vi "auto_sl.vi"() -> ()   [LabVIEW 2012, in "Serenity_mk2.lvrbt"]
uses:
  Serenity_mk2.lvrbt
  MecanumDrive/Mecanum Drive.lvrbt
  <vilib>/NXT/Hardware/Plugins/Tetrix DC Motor/TetrixDCMotorAddress.ctl
  <vilib>/NXT/LegoClasses/BrickReference/BrickReference.lvclass
  <vilib>/NXT/Subs/LVHSConnector.ctl
  <vilib>/NXT/NXTIO Xnodes/NXTIONodeSubVIs/TETRIX IO Stop DC Motors.vi
  <vilib>/NXT/NXTIO Xnodes/NXTIOXNode/NXTIO.xnode
  <vilib>/NXT/NXTIO Xnodes/AddressXNode/NXTIOAddress.xnode
  <vilib>/NXT/Block Support/NXT_InputPort.ctl
  <vilib>/NXT/HiTechnic/HiTechnic Controls/HiTechnic Port.ctl
  Serenity_mk2/SubVIs/State_Typ.ctl
  Serenity_mk2/SubVIs/auto_drive_TYP.ctl
  <vilib>/NXT/Dual Mode Library/Sound/Tone.vi
  <vilib>/NXT/Dual Mode Library/Waits/Wait_Num.vi
  <vilib>/NXT/Dual Mode Library/Display/drawNumber.vi
  <vilib>/NXT/Dual Mode Library/Waits/Wait_Num(msec).vi
  <vilib>/NXT/NXTIO Xnodes/NXTIONodeSubVIs/TETRIX IO Check Battery.vi
  <vilib>/NXT/NXTIO Xnodes/NXTIONodeSubVIs/TETRIX IO Reset Encoders.vi
  <vilib>/NXT/NXTIO Xnodes/NXTIONodeSubVIs/TETRIX IO Motor Status.vi
  <vilib>/NXT/Hardware/Plugins/Tetrix 180 deg Servo/Tetrix180ServoAddress.ctl
  <vilib>/NXT/NXTIO Xnodes/NXTIONodeSubVIs/TETRIX IO Move Servos.vi
panel:
  out "Enabled":bool
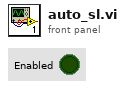
[diagram p1: front panel]
types:
  T1 = typedef "auto_drive_TYP.ctl" = cluster{"Left X":i8, "Left Y":i8, "Right X":i8, "Power (100)":i8, "Wait (ms)":u32, "Enc/Deg Target":i32, "Move Type":enum16{"Relative Degrees", "Wait", "Encoder"}}
  T2 = typedef "State_Typ.ctl" = enum16{"Stop", "Check for Position 3", "Check for Position 2", "Move", "Reset Enc", "Read Enc"}
  T3 = typedef "HiTechnic Port.ctl" = cluster{"Port":T4, "MUX Port":u8}
  T4 = typedef "NXT_InputPort.ctl" = u32
  T5 = typedef "TetrixDCMotorAddress.ctl" = i32
  T6 = typedef "LVHSConnector.ctl" = refnum<class "BrickReference.lvclass">
  T7 = typedef "Tetrix180ServoAddress.ctl" = i32
  T8 = cluster{"TetrixDCMotor":T5, "TetrixDCMotor 2":T5}
  T9 = cluster{"Direction (0-9)":i16, "Signal Strength (Array)":u8[]}
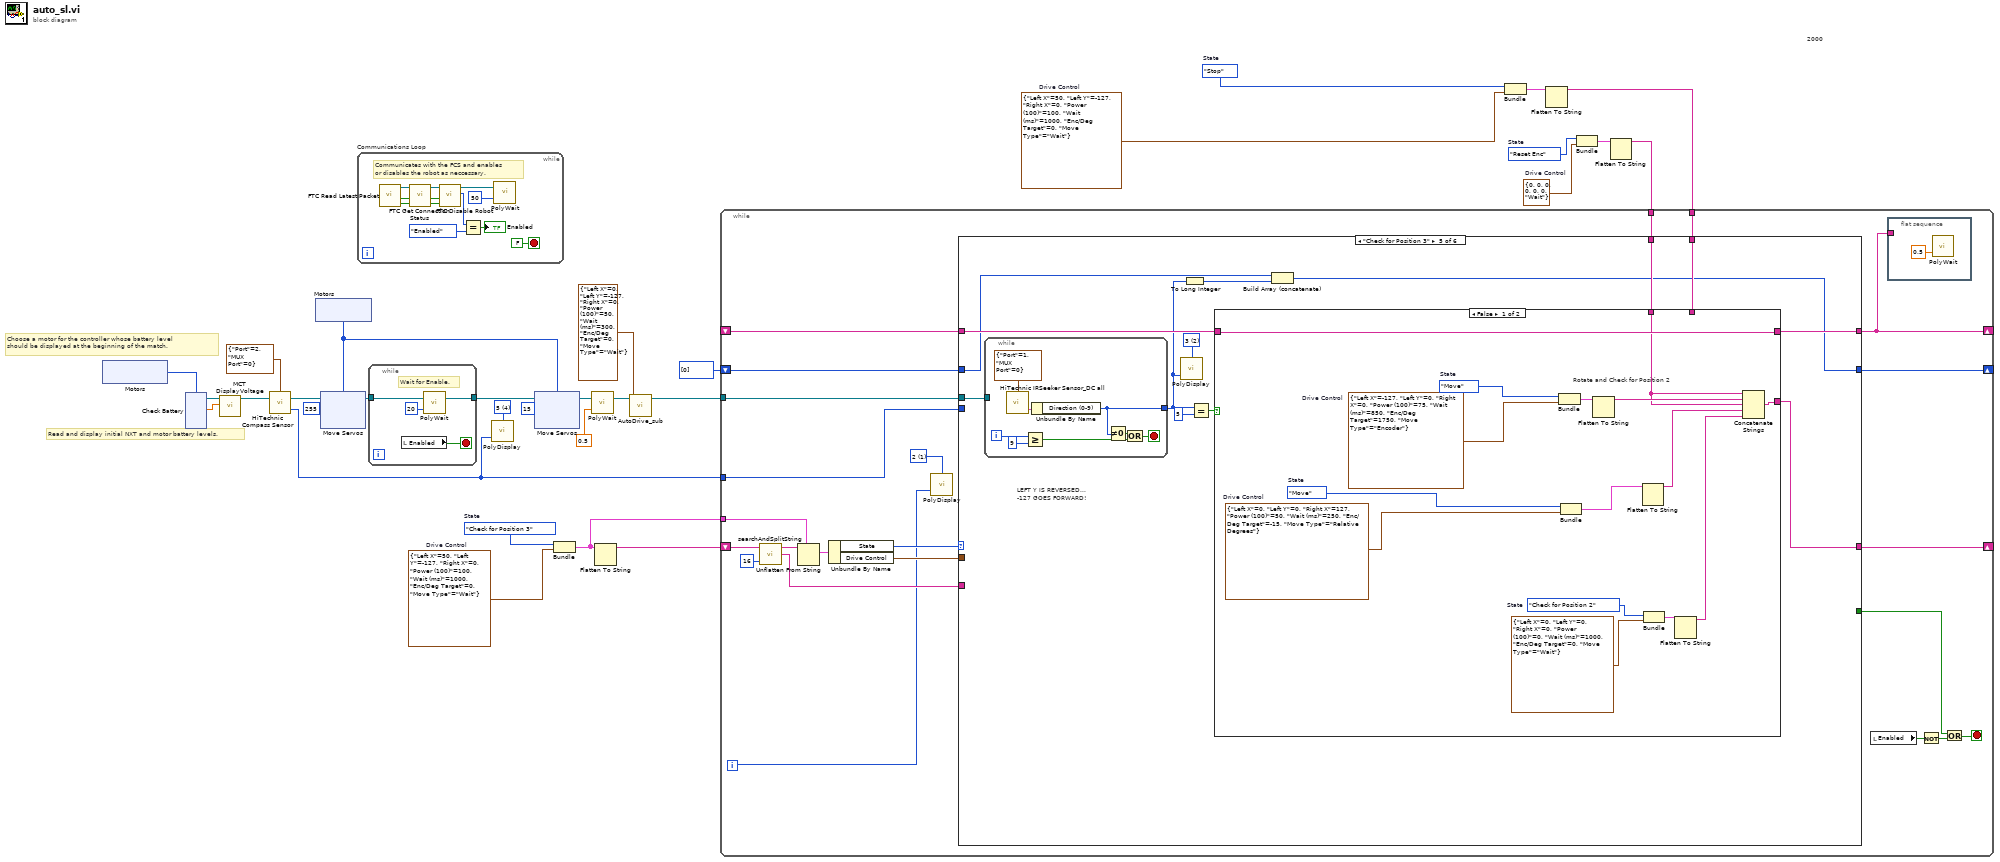
[diagram p0: block diagram]
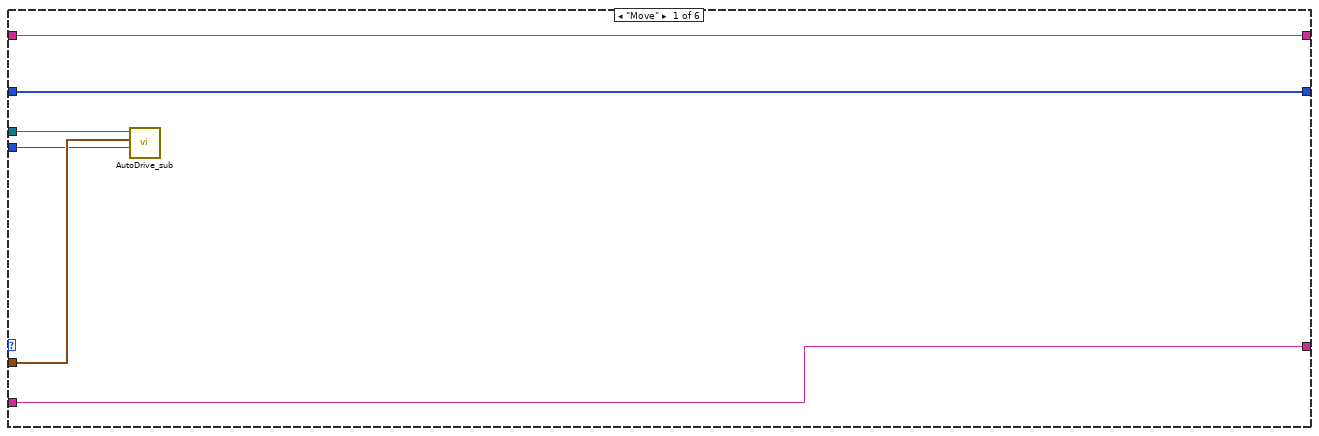
[diagram p2: hidden frame]
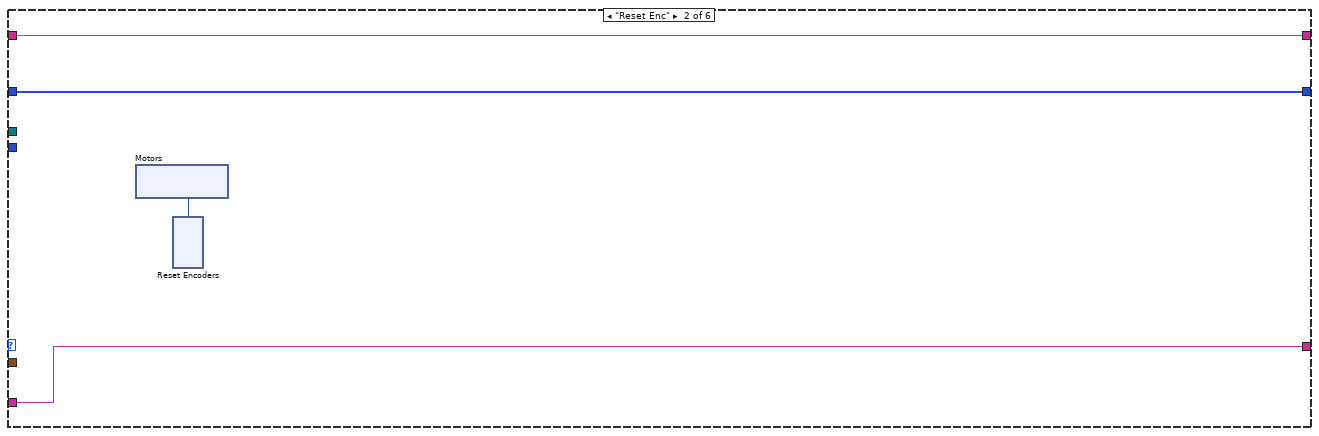
[diagram p3: hidden frame]
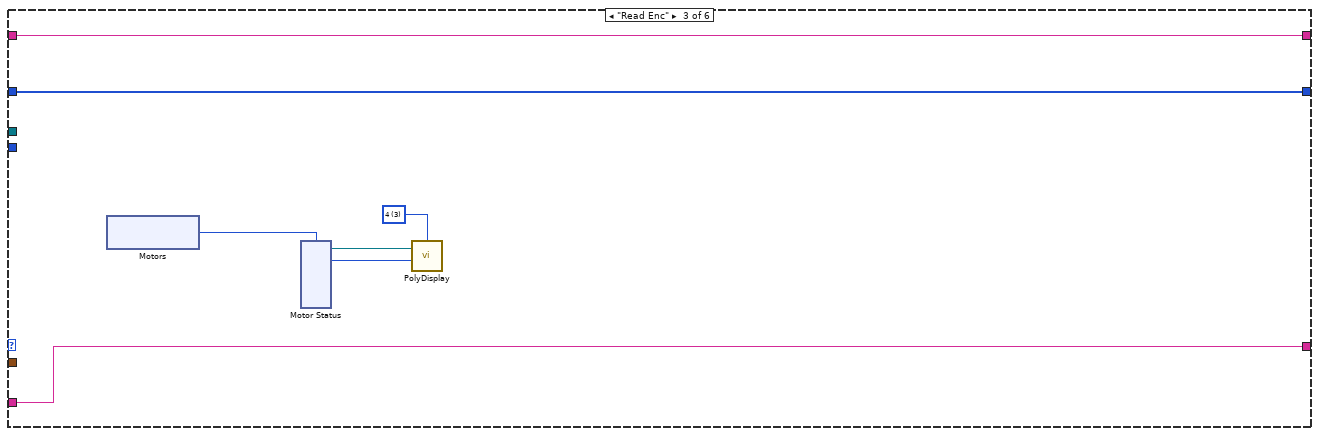
[diagram p4: hidden frame]
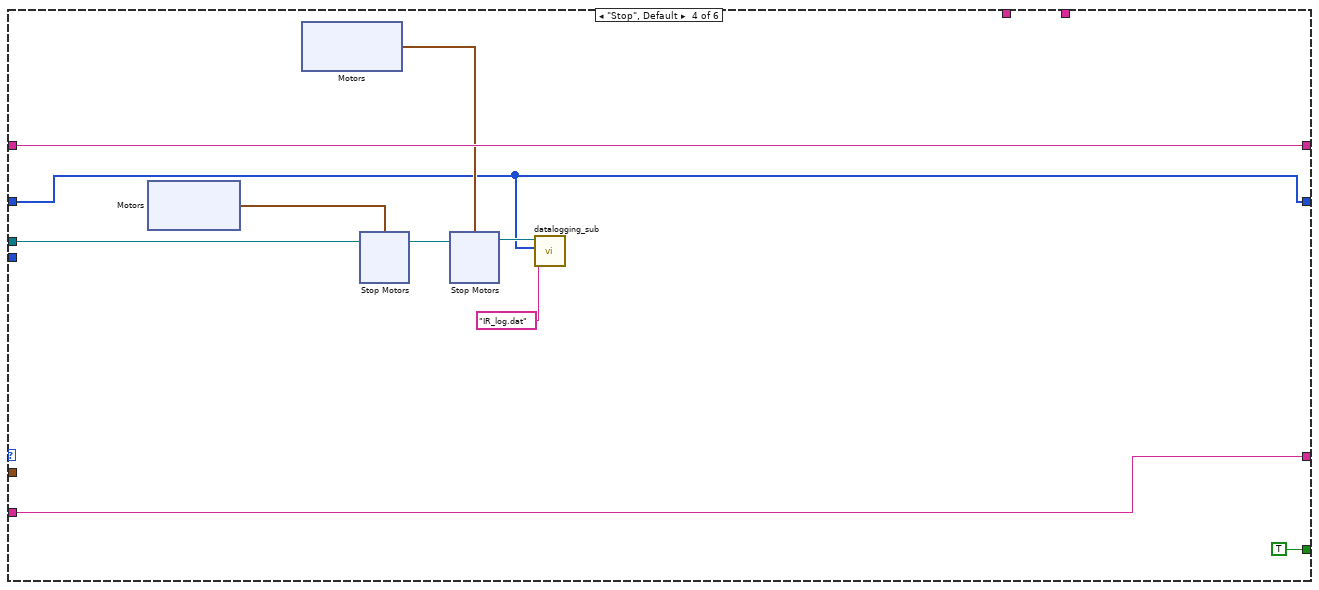
[diagram p5: hidden frame]
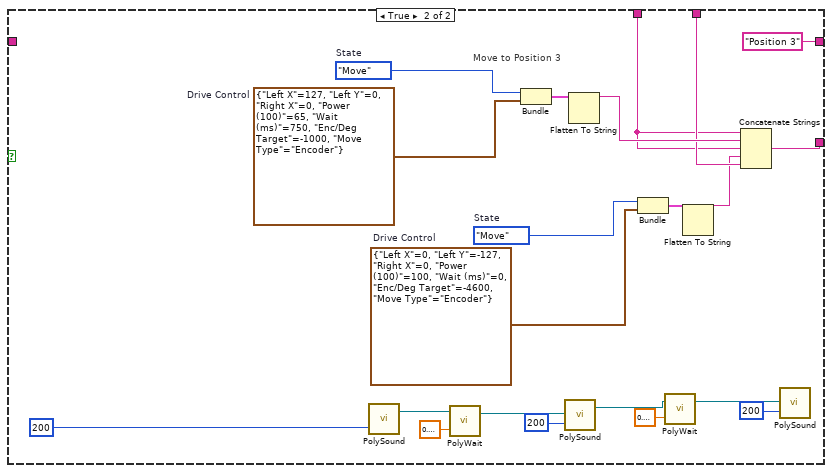
[diagram p6: hidden frame]
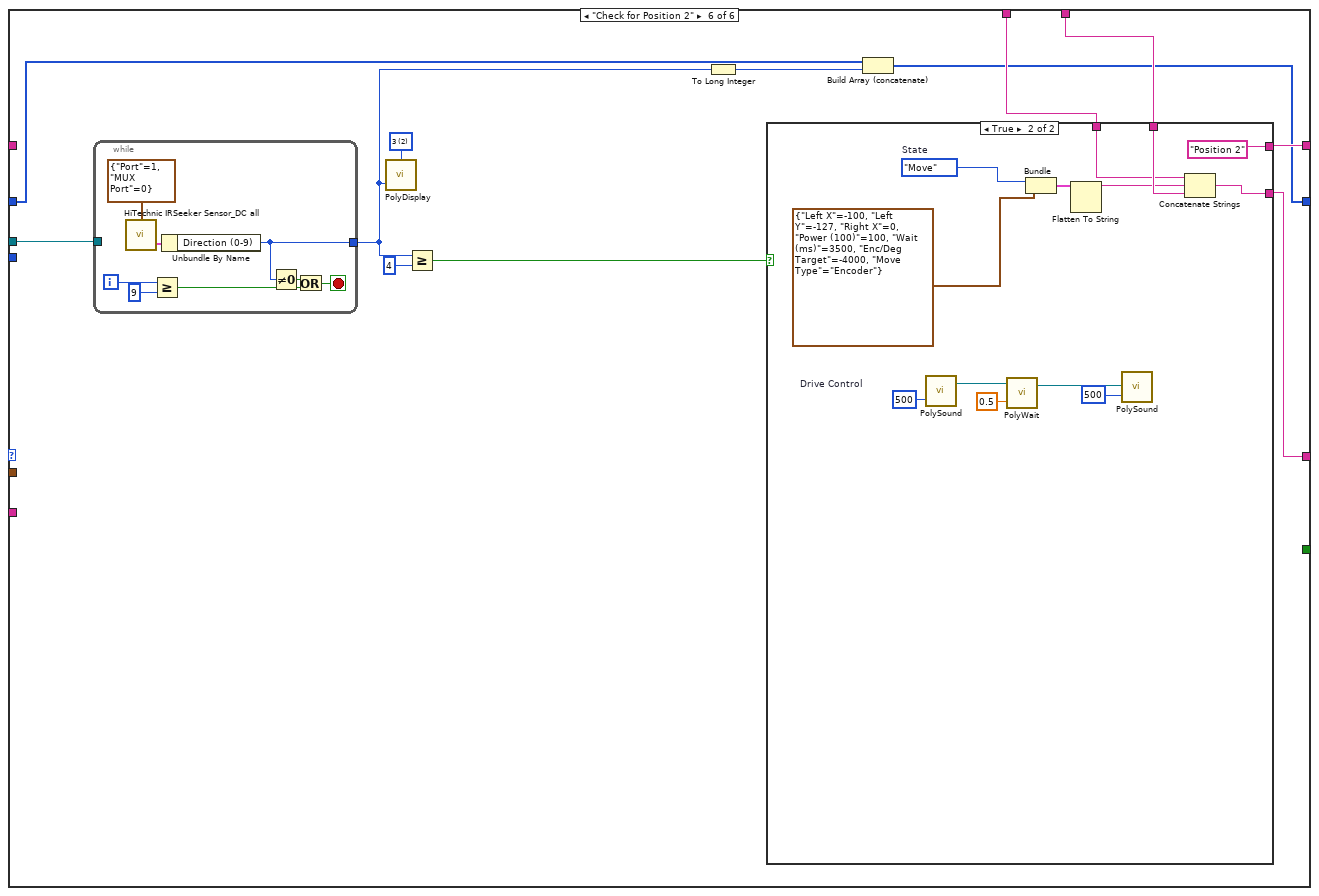
[diagram p7: hidden frame]
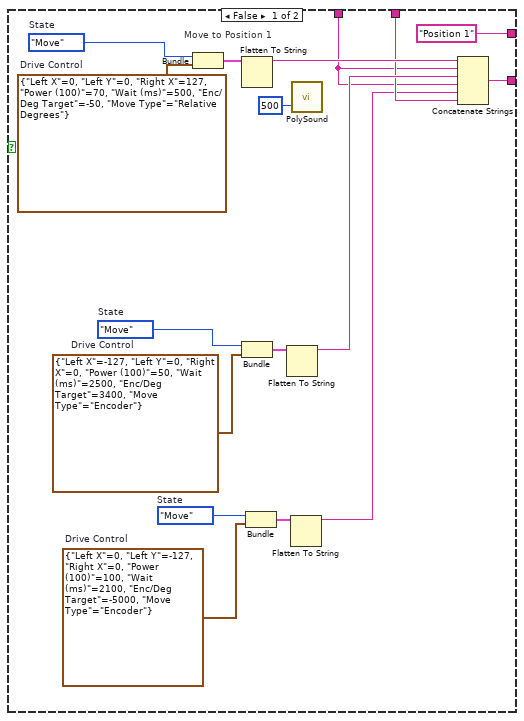
[diagram p8: hidden frame]
diagram:
  w11 = T1 {"Left X"=0, "Left Y"=0, "Right X"=0, "Power (100)"=0, "Wait (ms)"=0, "Enc/Deg Target"=0, "Move Type"=enum."Wait"}  # Drive Control
  w13 = State_Typ."Reset Enc"  # State
  w18 = T1 {"Left X"=50, "Left Y"=-127, "Right X"=0, "Power (100)"=100, "Wait (ms)"=1000, "Enc/Deg Target"=0, "Move Type"=enum."Wait"}  # Drive Control
  w19 = State_Typ."Stop"  # State
  w22 = i16 4 items=["1", "2", "3", "4", "5", "6", "7", "8", "9", "10", "11", "12"] ("Line")
  w31 = T1 {"Left X"=50, "Left Y"=-127, "Right X"=0, "Power (100)"=100, "Wait (ms)"=1000, "Enc/Deg Target"=0, "Move Type"=enum."Wait"}  # Drive Control
  w30 = State_Typ."Check for Position 3"  # State
  # "2000"
  # "Read and display initial NXT and motor battery levels."
  # "Choose a motor for the controller whose battery level \nshould be displayed at the beginning of the match."
  n1 = xnode "Motors"() -> ("Motor"=w27:T5)
  n2 = xnode "Check Battery"("Motors"=w27) -> ("Voltage 1"=w28:sgl, "NXT/EV3"=w29:T6)  [unwired: 1 in]
  n3 = call <vilib>:"MCT DisplayVoltage.vi"("Motor Voltage"=w28, "NXT"=w29) -> ("NXT"=w23:T6)  [unwired: 9 in]
  n4 = call <vilib>:"HiTechnic Compass Sensor.vi"("NXT/EV3"=w23, "Port/MUX"=T3 {"Port"=2, "MUX Port"=0}) -> ("Heading (degrees)"=w21:i16, "NXT/EV3"=w10:T6)  [unwired: 1 in]
  n5 = xnode "Motors"() -> ("Motor"=w6:T7)
  n6 = xnode "Move Servos"("Position 1"=u8 255, "Motors"=w6, "NXT/EV3"=w10) -> ("NXT/EV3"=w9:T6)
  n7 = while "Communications Loop" {
    stop <- FALSE stop-if-true
    # "Communicates with the FCS and enables \nor disables the robot as neccessary."
    n8 = call <vilib>:"FTC Read Latest Packet.vi"() -> ("Packet Received?"=w41:bool, "Stopped?"=w40:bool, "NXT"=w43:T6)  [unwired: 6 in, 3 out]
    n9 = call <vilib>:"FTC Get Connection Status.vi"("Packet Received?"=w41, "Stopped?"=w40, "NXT"=w43) -> ("Online?"=w32:bool, "Stopped?"=w33:bool, "NXT"=w42:T6)  [unwired: 5 in]
    n10 = call <vilib>:"FTC Disable Robot.vi"("Online?"=w32, "Stopped?"=w33, "NXT"=w42) -> ("Enabled?"=w36:enum16{"Disabled", "Enabled"}, "NXT"=w38:T6)  [unwired: 3 in]
    n11 = Equal?(x=w36, y=enum16{"Disabled", "Enabled"}."Enabled") -> (x = y?=→"Enabled":bool)
    n12 = call-poly <vilib>:"PolyWait.vi"("Time (100 msec)"=u32 50 ("Time (msec)"), "NXT/EV3"=w38) -> ()  [unwired: 2 in, 1 out]
  }
  n13 = while {
    tunnel: [w45] -> w5
    tunnel: w9 -> [w44]
    stop <- w46 stop-if-true
    # "Wait for Enable."
    n14 = local read "Enabled"() -> (w46:bool)
    n15 = call-poly <vilib>:"PolyWait.vi"("Time (100 msec)"=u32 20 ("Time (msec)"), "NXT/EV3"=w44) -> ("NXT/EV3"=w45:T6)  [unwired: 2 in]
  }
  n16 = call-poly <vilib>:"PolyDisplay.vi"("number"=w21, "Line"=w22) -> ()  [unwired: 2 in, 1 out]
  n17 = xnode "Move Servos"("Position 1"=u8 15, "Motors"=w6, "NXT/EV3"=w5) -> ("NXT/EV3"=w2:T6)
  n18 = Bundle("State"=w30, "Drive Control"=w31) -> (w26:cluster{"State":T2, "Drive Control":T1})  [unwired: 1 in]
  n19 = call-poly <vilib>:"PolyWait.vi"("Time (1 sec)"=sgl 0.5, "NXT/EV3"=w2) -> ("NXT/EV3"=w3:T6)  [unwired: 2 in]
  n20 = Flatten To String(anything=w26) -> (data string=w25:string)  [unwired: 3 in, 2 out]
  n21 = call "AutoDrive_sub.vi"("Drive Control"=T1 {"Left X"=0, "Left Y"=-127, "Right X"=0, "Power (100)"=50, "Wait (ms)"=300, "Enc/Deg Target"=0, "Move Type"=enum."Wait"}, "NXT/EV3"=w3) -> ("NXT/EV3 out"=w7:T6)  [unwired: 8 in, 1 out]
  n22 = Bundle("State"=w19, "Drive Control"=w18) -> (w20:cluster{"State":T2, "Drive Control":T1})  [unwired: 1 in]
  n23 = Flatten To String(anything=w20) -> (data string=w17:string)  [unwired: 3 in, 2 out]
  n24 = Bundle("State"=w13, "Drive Control"=w11) -> (w14:cluster{"State":T2, "Drive Control":T1})  [unwired: 1 in]
  n25 = Flatten To String(anything=w14) -> (data string=w12:string)  [unwired: 3 in, 2 out]
  n26 = while {
    tunnel: w7 -> [w70]
    shift-right: [w61] -> _
    shift-left: w25 -> [w59]
    tunnel: w26 -> [w62]
    shift-right: [w52] -> _
    shift-left: _ -> [w60]
    tunnel: w17 -> [w57]
    tunnel: w21 -> [w51]
    shift-right: [w50] -> _
    shift-left: i32[] [0] -> [w49]
    tunnel: w12 -> [w48]
    i -> [w53]
    stop <- w69 stop-if-true
    w54 = i16 1 items=["1", "2", "3", "4", "5", "6", "7", "8", "9", "10", "11", "12"] ("Line")
    n27 = call <vilib>:"searchAndSplitString.vi"("offset (0)"=16 ("length (rest)"), "string"=w59) -> ("match + rest of string"=w58:string, "substring before match"=w64:string)  [unwired: 1 in, 1 out]
    n28 = Unflatten From String(type=w62, binary string=w64) -> (value=w63:cluster{"State":T2, "Drive Control":T1})  [unwired: 3 in, 2 out]
    n29 = Unbundle By Name(w63) -> ("State"=w55:T2, "Drive Control"=w65:T1)
    n30 = call-poly <vilib>:"PolyDisplay.vi"("number"=w53, "Line"=w54) -> ()  [unwired: 2 in, 1 out]
    n31 = case shown="\"Check for Position 3\"" w55 {
      tunnel: w70 -> [w77 _ _ w112 w125 w186]
      tunnel: [_ _ _ TRUE _ _] -> w68
      tunnel: w65 -> [w76 _ _ _ _ _]
      tunnel: w58 -> [w75 w81 w93 w110 _ _]
      tunnel: [w75 w81 w93 w110 w133 w191] -> w61
      tunnel: [w74 w80 w92 w109 w136 w193] -> w52
      tunnel: w60 -> [w74 w80 w92 w109 w135 _]
      tunnel: w57 -> [_ _ _ _ w134 w192]
      tunnel: w51 -> [w73 _ _ _ _ _]
      tunnel: [w72 w78 w87 w104 w128 w189] -> w50
      tunnel: w49 -> [w72 w78 w87 w104 w129 w188]
      tunnel: w48 -> [_ _ _ _ w130 w190]
      frame "Move" {
        n32 = call "AutoDrive_sub.vi"("Target Heading (Degrees)"=w73, "Drive Control"=w76, "NXT/EV3"=w77) -> ()  [unwired: 7 in, 2 out]
      }
      frame "Reset Enc" {
        n33 = xnode "Motors"() -> ("Motor"=w79:T5)
        n34 = xnode "Reset Encoders"("Motors"=w79) -> ()  [unwired: 1 in, 1 out]
      }
      frame "Read Enc" {
        w89 = i16 3 items=["1", "2", "3", "4", "5", "6", "7", "8", "9", "10", "11", "12"] ("Line")
        n35 = xnode "Motors"() -> ("Motor"=w91:T5)
        n36 = xnode "Motor Status"("Motors"=w91) -> ("Position 1"=w90:i32, "NXT/EV3"=w88:T6)  [unwired: 1 in, 1 out]
        n37 = call-poly <vilib>:"PolyDisplay.vi"("number"=w90, "NXT/EV3"=w88, "Line"=w89) -> ()  [unwired: 1 in, 1 out]
      }
      frame "Stop", Default {
        n38 = xnode "Motors"() -> ("Motor"=w108:cluster{"TetrixDCMotor":T5, "TetrixDCMotor":T5})
        n39 = xnode "Motors"() -> ("Motor"=w107:cluster{"TetrixDCMotor":T5, "TetrixDCMotor":T5})
        n40 = xnode "Stop Motors"("Motors"=w108, "NXT/EV3"=w112) -> ("NXT/EV3"=w106:T6)
        n41 = xnode "Stop Motors"("Motors"=w107, "NXT/EV3"=w106) -> ("NXT/EV3"=w105:T6)
        n42 = call "datalogging_sub.vi"("Path Selected"="IR_log.dat" ("Filename"), "States Executed"=w104, "NXT/EV3 In"=w105) -> ()  [unwired: 8 in, 1 out]
      }
      frame "Check for Position 3" {
        w132 = i16 2 items=["1", "2", "3", "4", "5", "6", "7", "8", "9", "10", "11", "12"] ("Line")
        # "LEFT Y IS REVERSED...\n-127 GOES FORWARD!"
        n43 = while {
          tunnel: w125 -> [_]
          tunnel: [w143] -> w127
          i -> [w141]
          stop <- w138 stop-if-true
          n44 = call <vilib>:"HiTechnic IRSeeker Sensor_DC all.vi"("Port/MUX"=T3 {"Port"=1, "MUX Port"=0}) -> ("All Info"=w145:T9)  [unwired: 2 in, 1 out]
          n45 = Greater Or Equal?(x=w141, y=9 ("x")) -> (x >= y?=w139:bool)
          n46 = Unbundle By Name(w145) -> ("Direction (0-9)"=w143:i16)
          n47 = Not Equal To 0?(x=w143) -> (x != 0?=w142:bool)
          n48 = Or(x=w142, y=w139) -> (x .or. y?=w138:bool)
        }
        n49 = call-poly <vilib>:"PolyDisplay.vi"("number"=w127, "Line"=w132) -> ()  [unwired: 2 in, 1 out]
        n50 = To Long Integer(number=w127) -> (32bit integer=w126:i32)
        n51 = Equal?(x=w127, y=i16 5) -> (x = y?=w131:bool)
        n52 = case shown="False" w131 {
          tunnel: [w158 w174] -> w133
          tunnel: [w157 "Position 3"] -> w136
          tunnel: w135 -> [w157 _]
          tunnel: w134 -> [_ w172]
          tunnel: w130 -> [w150 w161]
          frame False {
            w147 = State_Typ."Check for Position 2"  # State
            w153 = T1 {"Left X"=0, "Left Y"=0, "Right X"=127, "Power (100)"=50, "Wait (ms)"=250, "Enc/Deg Target"=-15, "Move Type"=enum."Relative Degrees"}  # Drive Control
            w154 = State_Typ."Move"  # State
            w156 = T1 {"Left X"=-127, "Left Y"=0, "Right X"=0, "Power (100)"=75, "Wait (ms)"=850, "Enc/Deg Target"=1750, "Move Type"=enum."Encoder"}  # Drive Control
            w159 = State_Typ."Move"  # State
            # "Rotate and Check for Position 2"
            n53 = Bundle("State"=w159, "Drive Control"=w156) -> (w160:cluster{"State":T2, "Drive Control":T1})  [unwired: 1 in]
            n54 = Bundle("State"=w154, "Drive Control"=w153) -> (w155:cluster{"State":T2, "Drive Control":T1})  [unwired: 1 in]
            n55 = Flatten To String(anything=w160) -> (data string=w151:string)  [unwired: 3 in, 2 out]
            n56 = Flatten To String(anything=w155) -> (data string=w152:string)  [unwired: 3 in, 2 out]
            n57 = Bundle("State"=w147, "Drive Control"=T1 {"Left X"=0, "Left Y"=0, "Right X"=0, "Power (100)"=0, "Wait (ms)"=1000, "Enc/Deg Target"=0, "Move Type"=enum."Wait"}) -> (w149:cluster{"State":T2, "Drive Control":T1})  [unwired: 1 in]
            n58 = Flatten To String(anything=w149) -> (data string=w146:string)  [unwired: 3 in, 2 out]
            n59 = Concatenate Strings(w150, w151, w150, w152, w146) -> (w158:string)
          }
          frame True {
            w178 = T1 {"Left X"=0, "Left Y"=-127, "Right X"=0, "Power (100)"=100, "Wait (ms)"=0, "Enc/Deg Target"=-4600, "Move Type"=enum."Encoder"}  # Drive Control
            w179 = State_Typ."Move"  # State
            w181 = T1 {"Left X"=127, "Left Y"=0, "Right X"=0, "Power (100)"=65, "Wait (ms)"=750, "Enc/Deg Target"=-1000, "Move Type"=enum."Encoder"}  # Drive Control
            w180 = State_Typ."Move"  # State
            # "Move to Position 3"
            n60 = call-poly <vilib>:"PolySound.vi"("Duration (500 ms)"=u16 200) -> ("NXT/EV3"=w168:T6)  [unwired: 3 in]
            n61 = call-poly <vilib>:"PolyWait.vi"("Time (1 sec)"=sgl 0.2, "NXT/EV3"=w168) -> ("NXT/EV3"=w167:T6)  [unwired: 2 in]
            n62 = Bundle("State"=w180, "Drive Control"=w181) -> (w177:cluster{"State":T2, "Drive Control":T1})  [unwired: 1 in]
            n63 = call-poly <vilib>:"PolySound.vi"("Duration (500 ms)"=u16 200, "NXT/EV3"=w167) -> ("NXT/EV3"=w164:T6)  [unwired: 2 in]
            n64 = Flatten To String(anything=w177) -> (data string=w175:string)  [unwired: 3 in, 2 out]
            n65 = Bundle("State"=w179, "Drive Control"=w178) -> (w176:cluster{"State":T2, "Drive Control":T1})  [unwired: 1 in]
            n66 = call-poly <vilib>:"PolyWait.vi"("Time (1 sec)"=sgl 0.2, "NXT/EV3"=w164) -> ("NXT/EV3"=w163:T6)  [unwired: 2 in]
            n67 = Flatten To String(anything=w176) -> (data string=w162:string)  [unwired: 3 in, 2 out]
            n68 = Concatenate Strings(w161, w175, w161, w162, w172) -> (w174:string)
            n69 = call-poly <vilib>:"PolySound.vi"("Duration (500 ms)"=u16 200, "NXT/EV3"=w163) -> ()  [unwired: 2 in, 1 out]
          }
        }
        n70 = Build Array (concatenate)(w129, w126) -> (w128:i32[])
      }
      frame "Check for Position 2" {
        w184 = i16 2 items=["1", "2", "3", "4", "5", "6", "7", "8", "9", "10", "11", "12"] ("Line")
        n71 = while {
          tunnel: [w199] -> w182
          tunnel: w186 -> [_]
          i -> [w197]
          stop <- w194 stop-if-true
          n72 = call <vilib>:"HiTechnic IRSeeker Sensor_DC all.vi"("Port/MUX"=T3 {"Port"=1, "MUX Port"=0}) -> ("All Info"=w201:T9)  [unwired: 2 in, 1 out]
          n73 = Greater Or Equal?(x=w197, y=9 ("x")) -> (x >= y?=w195:bool)
          n74 = Unbundle By Name(w201) -> ("Direction (0-9)"=w199:i16)
          n75 = Not Equal To 0?(x=w199) -> (x != 0?=w198:bool)
          n76 = Or(x=w198, y=w195) -> (x .or. y?=w194:bool)
        }
        n77 = call-poly <vilib>:"PolyDisplay.vi"("number"=w182, "Line"=w184) -> ()  [unwired: 2 in, 1 out]
        n78 = Greater Or Equal?(x=w182, y=i16 4) -> (x >= y?=w183:bool)
        n79 = To Long Integer(number=w182) -> (32bit integer=w187:i32)
        n80 = case shown="True" w183 {
          tunnel: [w215 w228] -> w191
          tunnel: ["Position 1" "Position 2"] -> w193
          tunnel: w192 -> [w207 w221]
          tunnel: w190 -> [w202 w219]
          frame False {
            w205 = T1 {"Left X"=0, "Left Y"=-127, "Right X"=0, "Power (100)"=100, "Wait (ms)"=2100, "Enc/Deg Target"=-5000, "Move Type"=enum."Encoder"}  # Drive Control
            w206 = State_Typ."Move"  # State
            w213 = T1 {"Left X"=-127, "Left Y"=0, "Right X"=0, "Power (100)"=50, "Wait (ms)"=2500, "Enc/Deg Target"=3400, "Move Type"=enum."Encoder"}  # Drive Control
            w214 = State_Typ."Move"  # State
            w217 = T1 {"Left X"=0, "Left Y"=0, "Right X"=127, "Power (100)"=70, "Wait (ms)"=500, "Enc/Deg Target"=-50, "Move Type"=enum."Relative Degrees"}  # Drive Control
            w218 = State_Typ."Move"  # State
            # "Move to Position 1"
            n81 = Bundle("State"=w218, "Drive Control"=w217) -> (w216:cluster{"State":T2, "Drive Control":T1})  [unwired: 1 in]
            n82 = Flatten To String(anything=w216) -> (data string=w209:string)  [unwired: 3 in, 2 out]
            n83 = Bundle("State"=w214, "Drive Control"=w213) -> (w212:cluster{"State":T2, "Drive Control":T1})  [unwired: 1 in]
            n84 = Bundle("State"=w206, "Drive Control"=w205) -> (w204:cluster{"State":T2, "Drive Control":T1})  [unwired: 1 in]
            n85 = Flatten To String(anything=w212) -> (data string=w211:string)  [unwired: 3 in, 2 out]
            n86 = Flatten To String(anything=w204) -> (data string=w203:string)  [unwired: 3 in, 2 out]
            n87 = call-poly <vilib>:"PolySound.vi"("Duration (500 ms)"=u16 500) -> ()  [unwired: 3 in, 1 out]
            n88 = Concatenate Strings(w209, w202, w211, w202, w203, w207) -> (w215:string)
          }
          frame True {
            w230 = T1 {"Left X"=-100, "Left Y"=-127, "Right X"=0, "Power (100)"=100, "Wait (ms)"=3500, "Enc/Deg Target"=-4000, "Move Type"=enum."Encoder"}  # Drive Control
            w229 = State_Typ."Move"  # State
            n89 = call-poly <vilib>:"PolySound.vi"("Duration (500 ms)"=u16 500) -> ("NXT/EV3"=w223:T6)  [unwired: 3 in]
            n90 = call-poly <vilib>:"PolyWait.vi"("Time (1 sec)"=sgl 0.5, "NXT/EV3"=w223) -> ("NXT/EV3"=w222:T6)  [unwired: 2 in]
            n91 = Bundle("State"=w229, "Drive Control"=w230) -> (w231:cluster{"State":T2, "Drive Control":T1})  [unwired: 1 in]
            n92 = Flatten To String(anything=w231) -> (data string=w220:string)  [unwired: 3 in, 2 out]
            n93 = call-poly <vilib>:"PolySound.vi"("Duration (500 ms)"=u16 500, "NXT/EV3"=w222) -> ()  [unwired: 2 in, 1 out]
            n94 = Concatenate Strings(w219, w220, w221) -> (w228:string)
          }
        }
        n95 = Build Array (concatenate)(w188, w187) -> (w189:i32[])
      }
    }
    n96 = local read "Enabled"() -> (w67:bool)
    n97 = flat-sequence {
      tunnel: w52 -> [_]
      frame #0 {
        n98 = call-poly <vilib>:"PolyWait.vi"("Time (1 sec)"=sgl 0.5) -> ()  [unwired: 3 in, 1 out]
      }
    }
    n99 = Not(x=w67) -> (.not. x?=w56:bool)
    n100 = Or(x=w68, y=w56) -> (x .or. y?=w69:bool)
  }
